vi "StartOneAxisHomeMove.vi"(8 "error in (no error)":errorcluster, 9 "mmWave Axis to Home":T1="BS1", 11 "VXMMotionManager in":refnum<class "VXMMotionManager.lvclass">) -> (0 "error out":errorcluster, 3 "VXMMotionManager out":refnum<class "VXMMotionManager.lvclass">)   [LabVIEW 2019, in "VXMMotionManager.lvclass"]
doc: "home just one axis.\nBe sure to move probe up out of the way and then back first.\nThis requires finding the current Z position in steps."
uses:
  VXMMotionManager.lvclass
  APARMainSubvis/VXM Public API/mmWaveAxis.ctl
  MoveAllAbsoluteStates.ctl
  APARMainSubvis/VXM Public API/singleAxisMoveDef.ctl
  VXMMotionManager.lvclass/VXMMotionManager.ctl
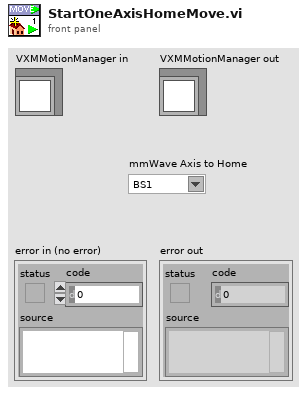
[diagram p1: front panel]
types:
  T1 = typedef "mmWaveAxis.ctl" = string
  T2 = typedef "singleAxisMoveDef.ctl" = cluster{"mmWave Axis":T1, "eng. value":dbl}
  T3 = typedef "VXMMotionManager.lvclass/MoveAllAbsoluteStates.ctl" = enum16{"start next move", "wait motion end"}
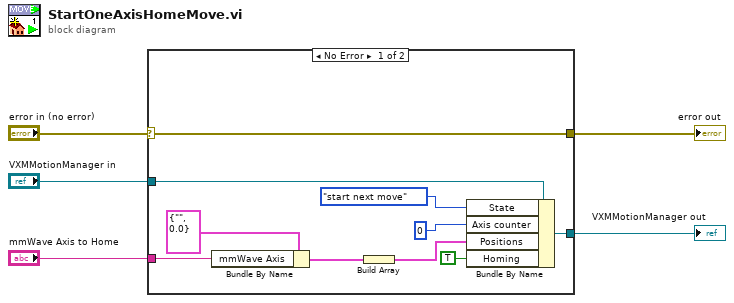
[diagram p0: block diagram]
diagram:
  n1 = case shown="No Error" "error in (no error)" {
    selector: "error in (no error)" -> [w15 w17]
    tunnel: [w15 w17] -> w4
    tunnel: [w13 w16] -> w2
    tunnel: "VXMMotionManager in" -> [w11 w16]
    tunnel: "mmWave Axis to Home" -> [w9 _]
    frame No Error {
      n2 = Bundle By Name(cluster=T2 {"mmWave Axis"="", "eng. value"=0.0} ("Move"), "mmWave Axis"=w9) -> (w8:T2)
      n3 = Build Array(w8) -> (w7:T2[])
      n4 = Bundle By Name(cluster=w11, "State"=MoveAllAbsoluteStates."start next move", "Axis counter"=0 ("Axis (0-3)"), "Positions"=w7, "Homing"=TRUE) -> (w13:refnum<class "VXMMotionManager.lvclass">)
    }
    frame Error {
    }
  }
  "error out" <- w4
  "VXMMotionManager out" <- w2
